vi "Load_McP_CounterPos.dat.vi"(0 "McP Counter Position Path":path) -> (1 "Counter Position":dbl=1620.34567 format="%.5f", 2 "Stepper Position":i32, 3 "Last Calibration Date":string=" 1620.34567\r")   [LabVIEW 2020]
panel:
  out "MCP Counter Position.dat path":path
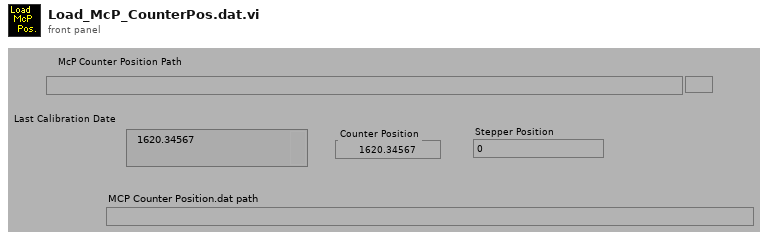
[diagram p1: front panel]
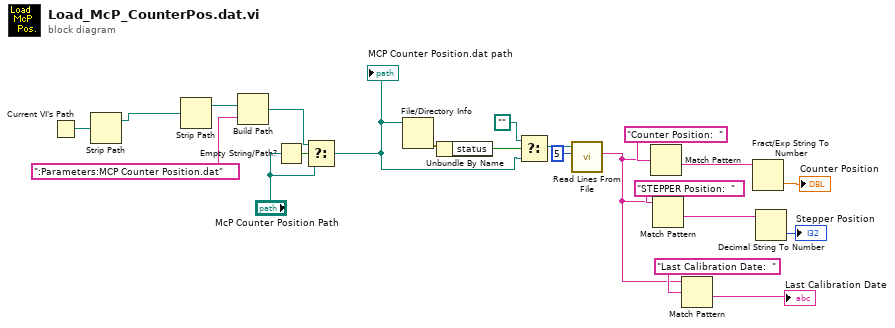
[diagram p0: block diagram]
diagram:
  n1 = Current VI's Path() -> (path=w4:path)
  n2 = Strip Path(path=w4) -> (stripped path=w1:path)  [unwired: 1 out]
  n3 = Strip Path(path=w1) -> (stripped path=w5:path)  [unwired: 1 out]
  n4 = Build Path(base path=w5, name or relative path=":Parameters:MCP Counter Position.dat") -> (appended path=w3:path)
  n5 = Empty String/Path?(string/path="McP Counter Position Path") -> (empty?=w8:bool)
  n6 = Select(t=w3, s=w8, f="McP Counter Position Path") -> (s? t:f=w2:path)
  "MCP Counter Position.dat path" <- w2
  n7 = File/Directory Info(path=w2) -> (error out=w12:errorcluster)  [unwired: 1 in, 6 out]
  n8 = Unbundle By Name(w12) -> ("status"=w11:bool)
  n9 = Select(t=path "", s=w11, f=w2) -> (s? t:f=w9:path)
  n10 = call <vilib>:"Read Lines From File.vi"("file path (dialog if empty)"=w9, "number of lines (all:-1)"=5) -> ("line string"=w14:string)  [unwired: 4 in, 3 out]
  n11 = Match Pattern(string=w14, regular expression="Counter Position:  ") -> (after substring=w16:string)  [unwired: 1 in, 3 out]
  n12 = Match Pattern(string=w14, regular expression="STEPPER Position:  ") -> (after substring=w13:string)  [unwired: 1 in, 3 out]
  n13 = Match Pattern(string=w14, regular expression="Last Calibration Date:  ") -> (after substring=→"Last Calibration Date":string)  [unwired: 1 in, 3 out]
  n14 = Fract/Exp String To Number(string=w16) -> (number=→"Counter Position":dbl)  [unwired: 3 in, 1 out]
  n15 = Decimal String To Number(string=w13) -> (number=→"Stepper Position":i32)  [unwired: 2 in, 1 out]
